vi "GVHorstSP.vi"() -> ()   [LabVIEW 2017]
panel:
  out "HorstSP":dbl[](array[numeric])
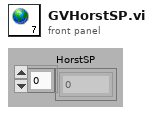
[diagram p1: front panel]
diagram:
